vi "Ball&Plate_PID.vi"() -> ()   [LabVIEW 2012]
uses:
  <vilib>/LabVIEW Interface for Arduino/Type Defs/Board Type.ctl
  <vilib>/addons/control/pid/pid.llb/PID (DBL).vi
  <vilib>/LabVIEW Interface for Arduino/LabVIEW Interface for Arduino.lvlib
  <vilib>/vision/NI_Vision_Development_Module.lvlib
  <vilib>/addons/control/pid/NI_PID_pid.lvlib
panel:
  out "Frame Rate":dbl
  out "Posicion actual vs Referencia":cluster{i32[], i32[]}[](graph)
  out "Posicion en el tiempo":cluster{i32, i32}[](graph)
  out "Respuesta en el tiempo":dynamicdata(graph)
  out "Salida PID Y":dbl format="%.2f"
  out "Salida Actuador Y":i32
  out "dt out (s) Y":dbl format="%.3f"
  in  "stop":bool
  in  "Tiempo De Muestreo (ms)":i32
  in  "reinitialize? (F)":bool
  out "dt out (s) X":dbl format="%.3f"
  in  "PID gains":T1={"proportional gain (Kc)"=1.0, "integral time (Ti, min)"=0.01, "derivative time (Td, min)"=0.0} {"derivative time (Td, min)" format="%.3f"; "integral time (Ti, min)" format="%.3f"; "proportional gain (Kc)" format="%.3f"}
  in  "output range":cluster{"output high":dbl, "output low":dbl}={"output high"=100.0, "output low"=-100.0} {"output low" format="%.2f"; "output high" format="%.2f"}
  out "Salida PID X":dbl
  out "ErrorY":dbl
  out "ErrorX":dbl
  in  "Baud Rate (115200)":u32=115200
  in  "Board Type (Uno)":T2
  in  "VISA resource":refnum<visa-resource-name>
  out "Salida Actuador X":i32
  in  "setpoint Y":i32
  in  "setpoint X":i32
  out "Ball and Plate":T3(plugin-control)
  out "POS(X)":i32
  out "POS(Y)":i32
  # "9"
  # "-9"
  # "CONSTANTES"
  # "KP\nKI\nKD"
  # "0,275"
  # "0,375"
  # "0,343"
  # "0,005"
  # "4,985"
  # "0,083"
  # "0,025"
  # "1,256"
  # "0,021"
  # "0,035"
  # "80"
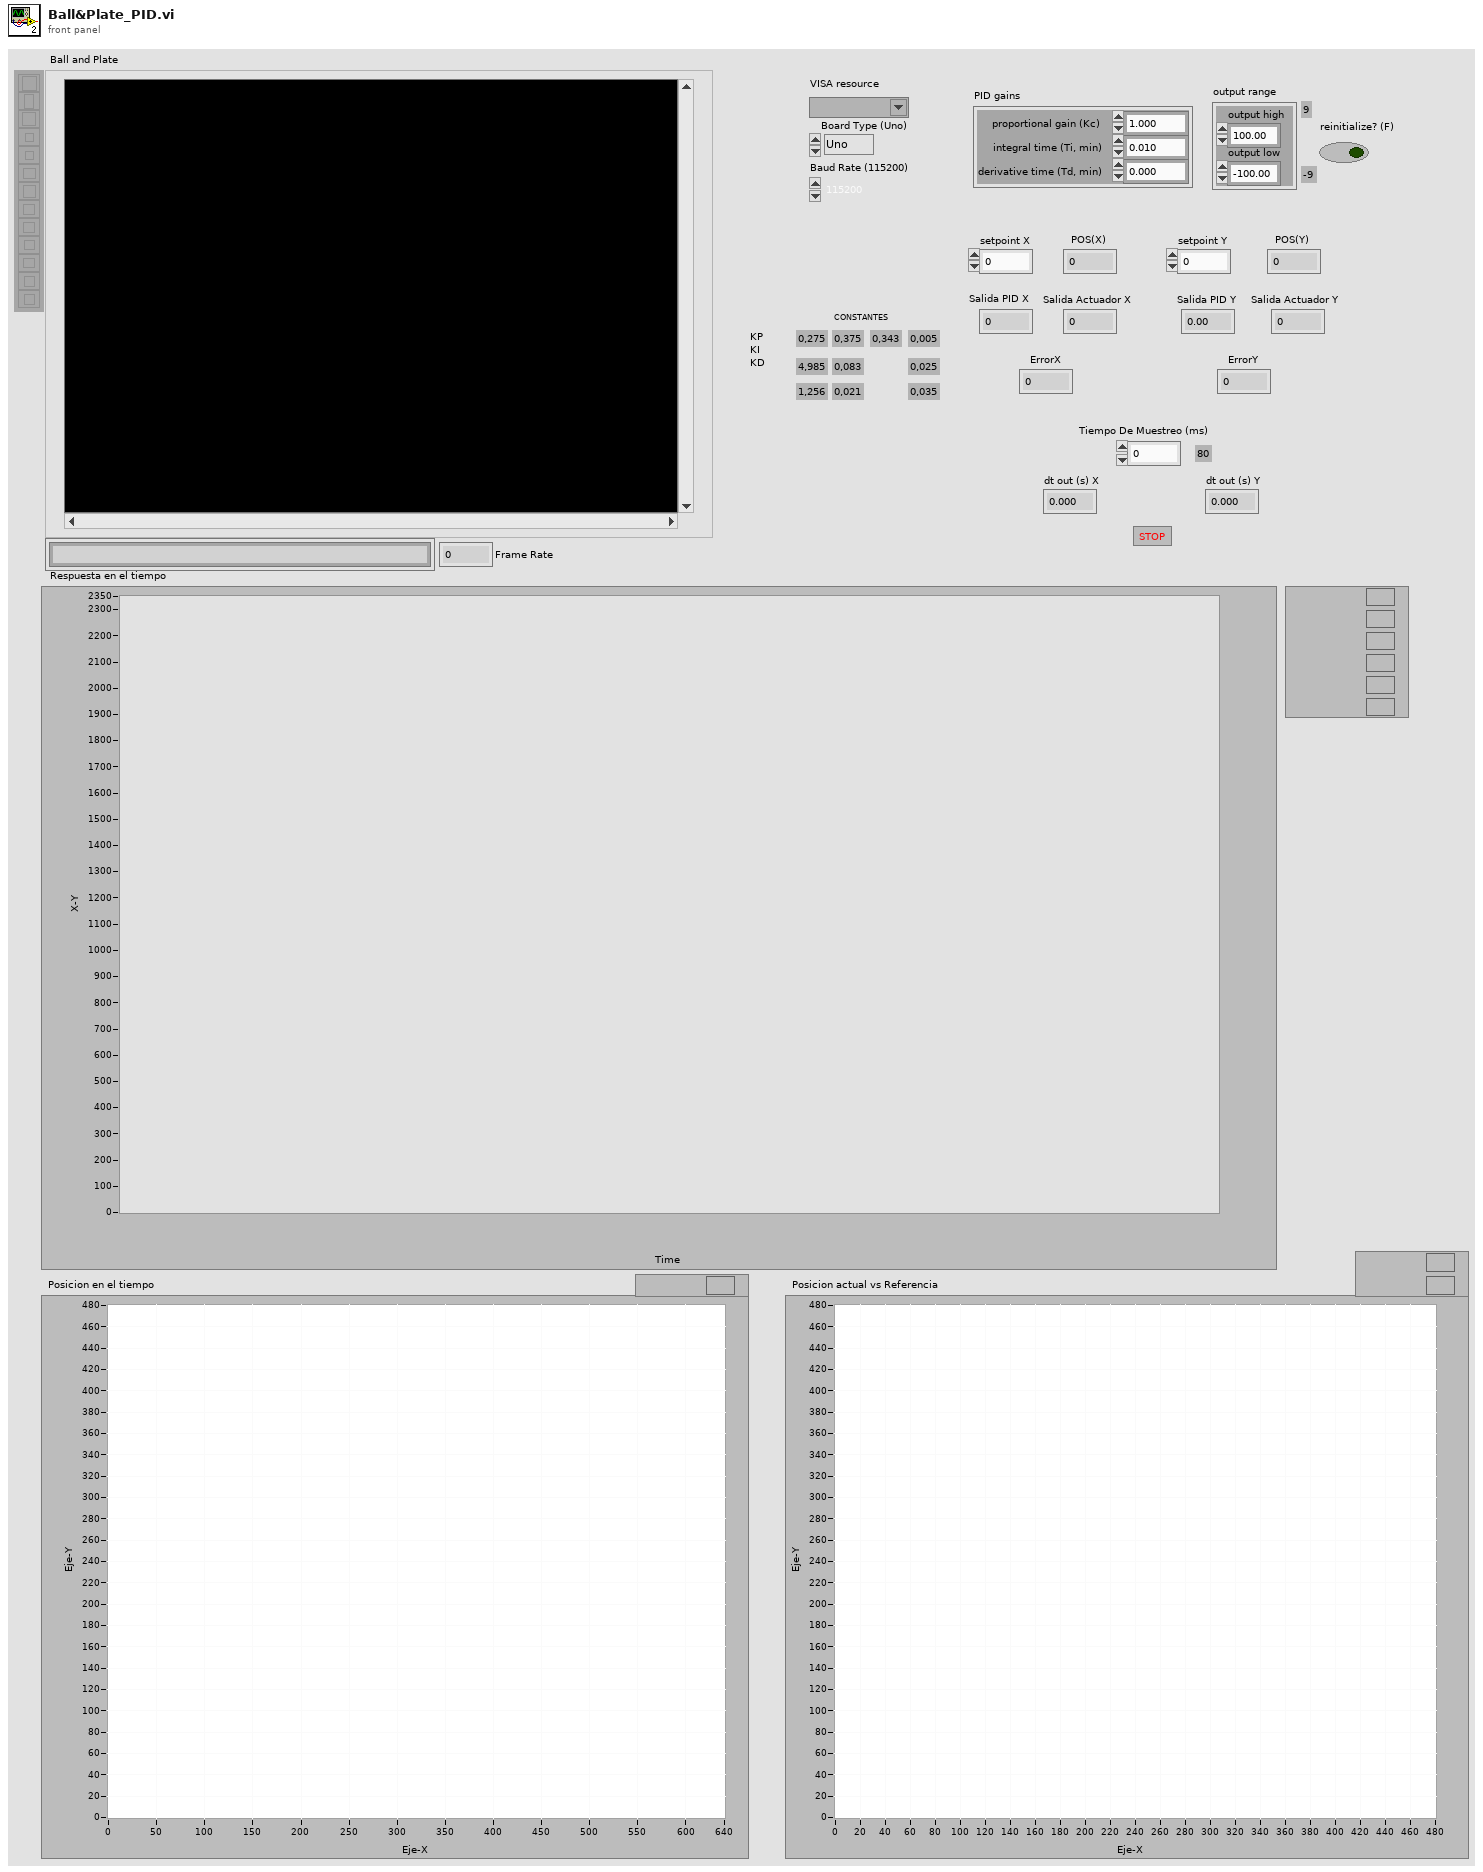
[diagram p1: front panel]
types:
  T1 = cluster{"proportional gain (Kc)":dbl, "integral time (Ti, min)":dbl, "derivative time (Td, min)":dbl}
  T2 = typedef "LabVIEW Interface for Arduino.lvlib/Board Type.ctl" = enum16{"Uno", "Dimuelanove w/Atmega 328", "Mega 2560"}
  T3 = typedef "IMAQ Image.ctl" = refnum<image>
  T4 = typedef "Image Type" = u32
  T5 = typedef "LabVIEW Interface for Arduino.lvlib/Arduino Resource.ctl" = cluster{"VISA resource":refnum<visa-resource-name>, "Board Type":T2, "Connection Type":enum8{"USB / Serial"}, "Bytes Per Packet (15)":u8}
  T6 = cluster{"Position":cluster{"x":sgl, "y":sgl}, "Angle":sgl, "Scale":sgl, "Score":sgl, "Bounding Box":cluster{"x":sgl, "y":sgl}[]}[]
  T7 = cluster{"Matches (Pattern Matching 1)[0]":cluster{"Position":cluster{"x":sgl, "y":sgl}, "Angle":sgl, "Scale":sgl, "Score":sgl, "Bounding Box":cluster{"x":sgl, "y":sgl}[]}, "Matches (Pattern Matching 1)[1]":cluster{"Position":cluster{"x":sgl, "y":sgl}, "Angle":sgl, "Scale":sgl, "Score":sgl, "Bounding Box":cluster{"x":sgl, "y":sgl}[]}, "Matches (Pattern Matching 1)[2]":cluster{"Position":cluster{"x":sgl, "y":sgl}, "Angle":sgl, "Scale":sgl, "Score":sgl, "Bounding Box":cluster{"x":sgl, "y":sgl}[]}, "Matches (Pattern Matching 1)[3]":cluster{"Position":cluster{"x":sgl, "y":sgl}, "Angle":sgl, "Scale":sgl, "Score":sgl, "Bounding Box":cluster{"x":sgl, "y":sgl}[]}}
  T8 = cluster{"Bounding Box[0]":cluster{"x":sgl, "y":sgl}, "Bounding Box[1]":cluster{"x":sgl, "y":sgl}, "Bounding Box[2]":cluster{"x":sgl, "y":sgl}, "Bounding Box[3]":cluster{"x":sgl, "y":sgl}}
  T9 = cluster{"[0]":sgl, "[1]":sgl, "[2]":sgl, "[3]":sgl}
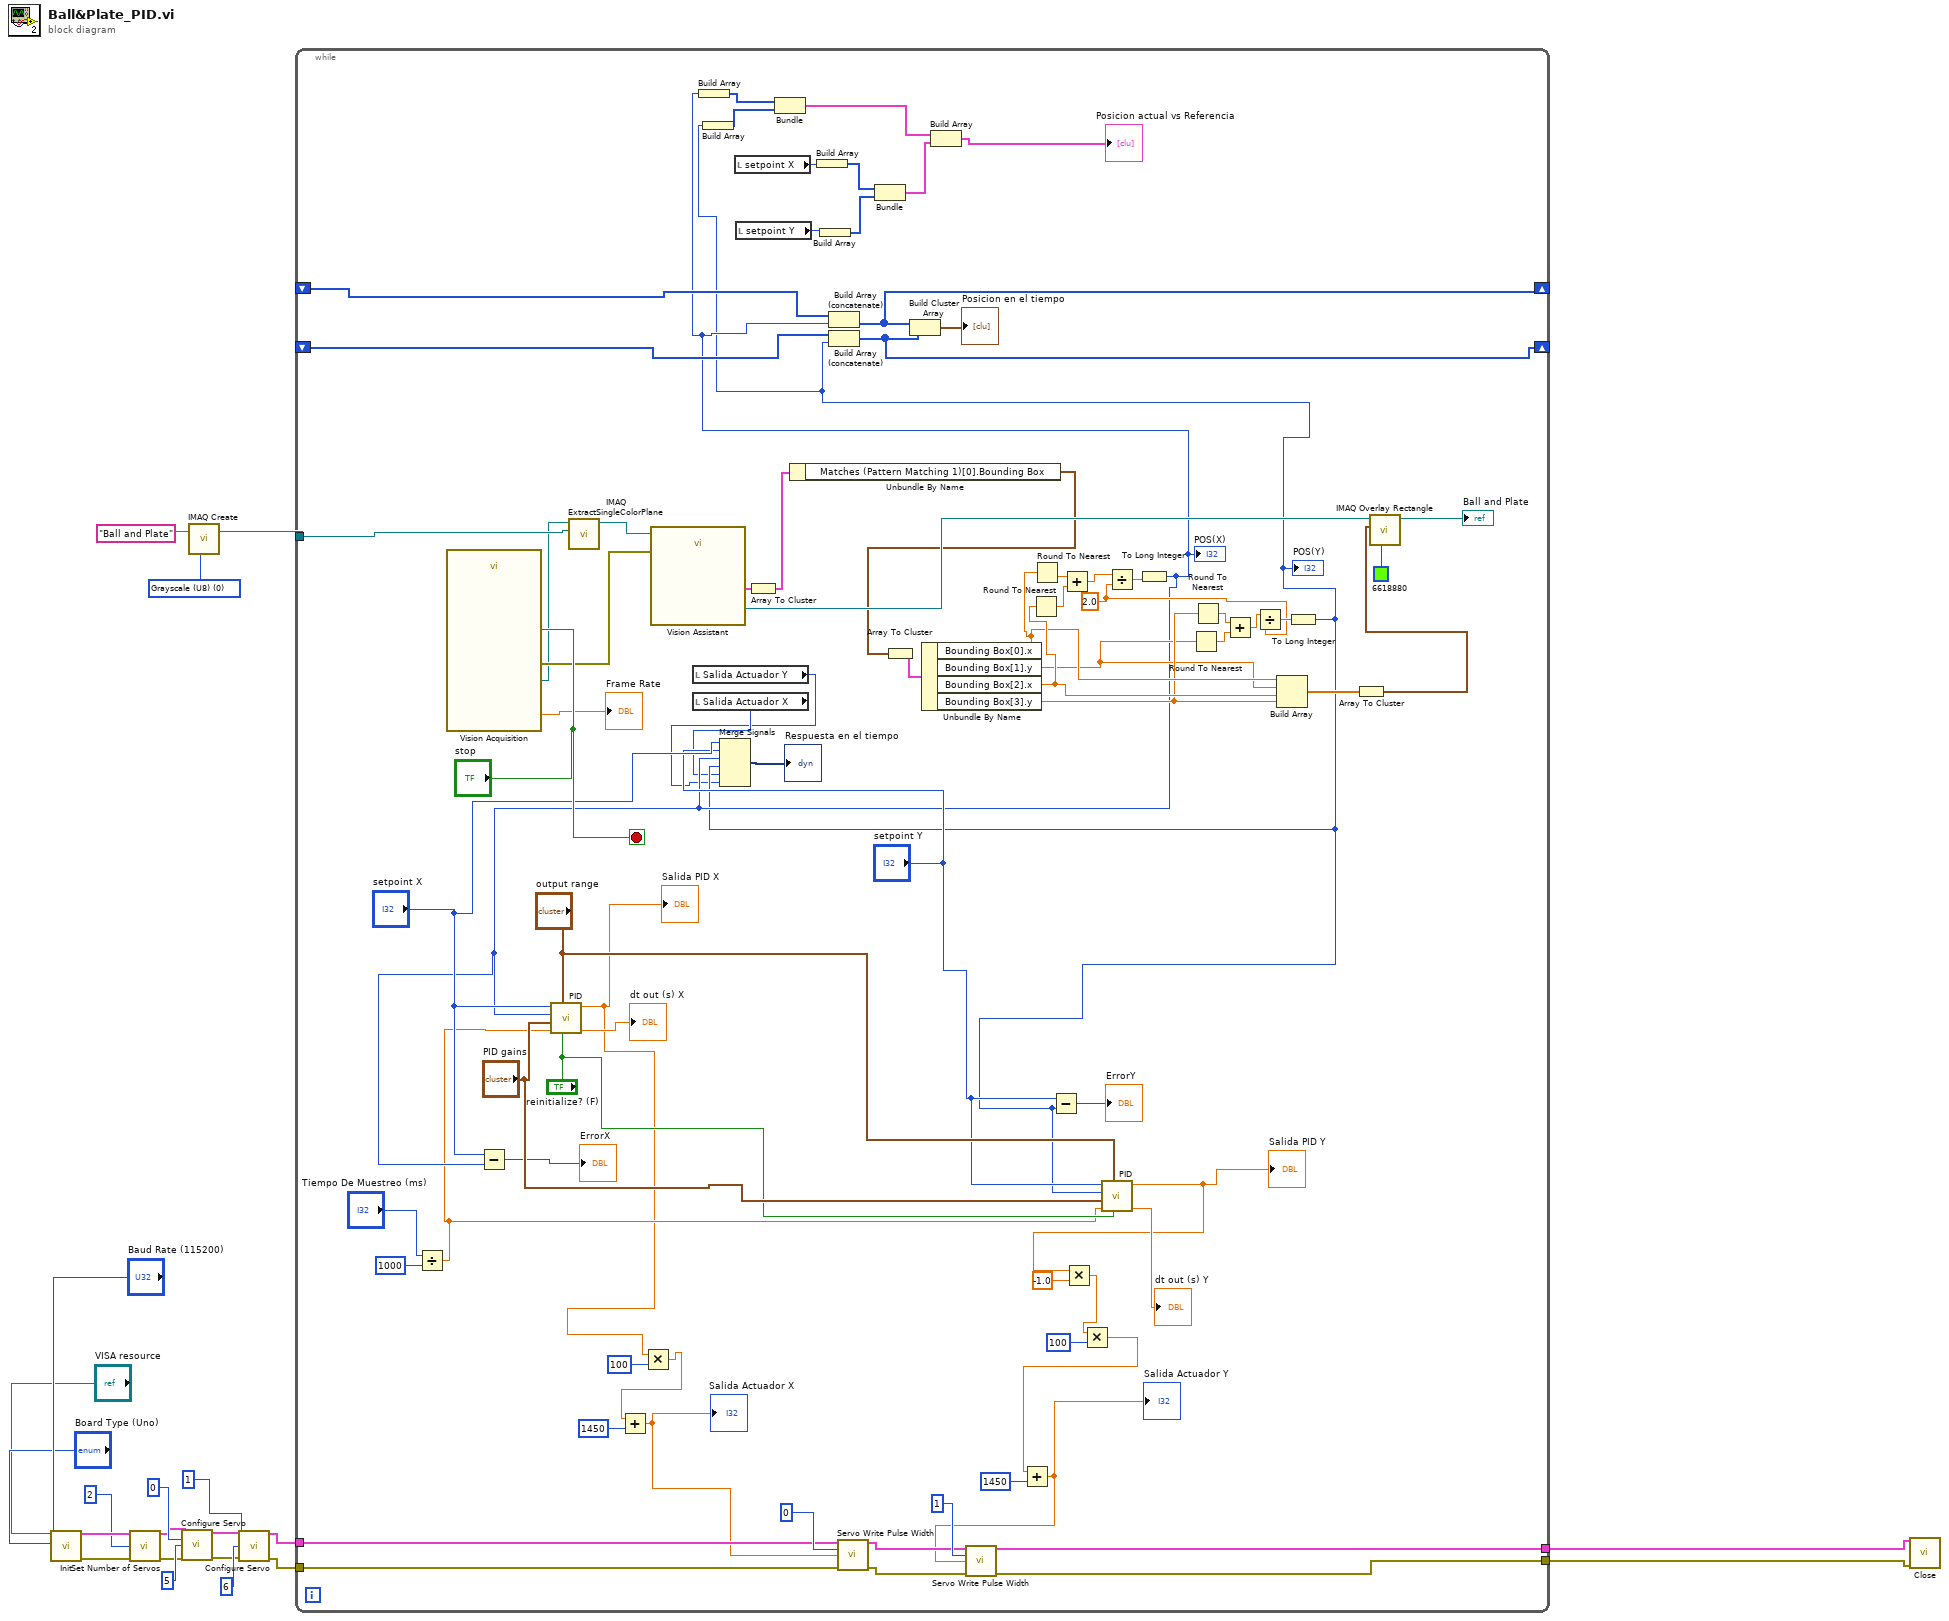
[diagram p0: block diagram]
diagram:
  w21 = T4 0 items=["Grayscale (U8)", "Grayscale (I16)", "Grayscale (SGL)", "Complex (CSG)", "RGB (U32)", "HSL (U32)", "RGB (U64)", "Grayscale (U16)"] ("Image Type")
  n1 = call <vilib>:"Init.vi"("VISA resource"="VISA resource", "Baud Rate (115200)"="Baud Rate (115200)", "Board Type (Uno)"="Board Type (Uno)") -> ("Arduino Resource"=w9:T5, "error out"=w8:errorcluster)  [unwired: 15 in]
  n2 = call <vilib>:"Set Number of Servos.vi"("Arduino Resource"=w9, "Number Of Servos (1)"=u8 2, "error in"=w8) -> ("Arduino Resource"=w10:T5, "error out"=w12:errorcluster)  [unwired: 11 in]
  n3 = call <vilib>:"Configure Servo.vi"("Arduino Resource"=w10, "Servo Number (0)"=u8 0, "DIO Pin (2)"=u8 5, "error in"=w12) -> ("Arduino Resource"=w11:T5, "error out"=w13:errorcluster)  [unwired: 10 in]
  n4 = call "IMAQ Create"("Image Name"="Ball and Plate", "Image Type"=w21) -> ("New Image"=w3:T3)  [unwired: 3 in, 1 out]
  n5 = call <vilib>:"Configure Servo.vi"("Arduino Resource"=w11, "Servo Number (0)"=u8 1, "DIO Pin (2)"=u8 6, "error in"=w13) -> ("Arduino Resource"=w5:T5, "error out"=w4:errorcluster)  [unwired: 10 in]
  n6 = while {
    tunnel: w5 -> [w95]
    tunnel: w4 -> [w94]
    tunnel: [w93] -> w2
    tunnel: w3 -> [w92]
    tunnel: [w58] -> w1
    shift-right: [w56] -> _
    shift-left: _ -> [w54]
    shift-right: [w55] -> _
    shift-left: _ -> [w53]
    stop <- "stop" stop-if-true
    w66 = sgl 2.0 ("x")
    n7 = Divide(x="Tiempo De Muestreo (ms)", y=1000) -> (x/y=w39:dbl)
    n8 = call "Vision Acquisition"("Stop (F)"="stop") -> ("Image Out"=w68:T3, "Frame Rate"=→"Frame Rate":dbl, "error out"=w75:errorcluster)  [unwired: 23 in, 1 out]
    n9 = call "IMAQ ExtractSingleColorPlane"("Image Dst"=w92, "Image Src"=w68) -> ("Image Dst Out"=w74:T3)  [unwired: 8 in, 1 out]
    n10 = call "Vision Assistant"("Image In"=w74, "error in"=w75) -> ("Image Out"=w77:T3, "Matches (Pattern Matching 1)"=w76:T6)  [unwired: 23 in, 1 out]
    n11 = local read "Salida Actuador Y"() -> (w26:i32)
    n12 = local read "Salida Actuador X"() -> (w27:i32)
    n13 = local read "setpoint X"() -> (w43:i32)
    n14 = local read "setpoint Y"() -> (w42:i32)
    n15 = Array To Cluster(array=w76) -> (cluster=w79:T7)
    n16 = Unbundle By Name(w79) -> ("Matches (Pattern Matching 1)[0].Bounding Box"=w71:cluster{"x":sgl, "y":sgl}[])
    n17 = Build Array(w43) -> (w52:i32[])
    n18 = Build Array(w42) -> (w51:i32[])
    n19 = Bundle(w52, w51) -> (w46:cluster{i32[], i32[]})  [unwired: 1 in]
    n20 = Array To Cluster ("Array To Cluster 2")(array=w71) -> (cluster=w72:T8)
    n21 = Unbundle By Name ("Unbundle By Name 2")(w72) -> ("Bounding Box[0].x"=w88:sgl, "Bounding Box[1].y"=w82:sgl, "Bounding Box[2].x"=w89:sgl, "Bounding Box[3].y"=w83:sgl)
    n22 = Round To Nearest(number=w89) -> (nearest integer value=w87:sgl)
    n23 = Round To Nearest ("Round To Nearest 3")(number=w88) -> (nearest integer value=w86:sgl)
    n24 = Add ("Add 2")(x=w86, y=w87) -> (x+y=w90:sgl)
    n25 = Divide(x=w90, y=w66) -> (x/y=w69:sgl)
    n26 = To Long Integer(number=w69) -> (32bit integer=w45:i32)
    "POS(X)" <- w45
    n27 = Subtract(x="setpoint X", y=w45) -> (x-y=→"ErrorX":i32)
    n28 = call-poly <vilib>:"PID.vi"("reinitialize? (F)"="reinitialize? (F)", "output range"="output range", "dt (s)"=w39, "PID gains"="PID gains", "process variable"=w45, "setpoint"="setpoint X") -> ("dt out (s)"=→"dt out (s) X":dbl, "output"=w36:dbl)  [unwired: 4 in]
    "Salida PID X" <- w36
    n29 = Multiply(x=w36, y=100) -> (x*y=w32:dbl)
    n30 = Add(x=w32, y=1450) -> (x+y=w23:dbl)
    "Salida Actuador X" <- w23
    n31 = Build Array(w45) -> (w50:i32[])
    n32 = Build Array (concatenate)(w54, w45) -> (w56:i32[])
    n33 = call <vilib>:"Servo Write Pulse Width.vi"("Arduino Resource"=w95, "Servo Number"=u8 0, "Pulse Width in uS"=w23, "error in"=w94) -> ("Arduino Resource"=w96:T5, "error out"=w97:errorcluster)  [unwired: 10 in]
    n34 = Round To Nearest ("Round To Nearest 2")(number=w82) -> (nearest integer value=w85:sgl)
    n35 = Round To Nearest ("Round To Nearest 4")(number=w83) -> (nearest integer value=w84:sgl)
    n36 = Add(x=w84, y=w85) -> (x+y=w67:sgl)
    n37 = Divide ("Divide 2")(x=w67, y=w66) -> (x/y=w70:sgl)
    n38 = Build Array(w88, w82, w89, w83) -> (w80:sgl[])
    n39 = To Long Integer(number=w70) -> (32bit integer=w44:i32)
    "POS(Y)" <- w44
    n40 = Build Array(w44) -> (w49:i32[])
    n41 = Merge Signals("setpoint X", "setpoint Y", w45, w44, w27, w26) -> (→"Respuesta en el tiempo":dynamicdata)
    n42 = Bundle(w50, w49) -> (w47:cluster{i32[], i32[]})  [unwired: 1 in]
    n43 = Build Array (concatenate)(w53, w44) -> (w55:i32[])
    n44 = Build Cluster Array(w56, w55) -> (→"Posicion en el tiempo":cluster{i32, i32}[])
    n45 = Build Array(w47, w46) -> (→"Posicion actual vs Referencia":cluster{i32[], i32[]}[])
    n46 = Subtract ("Subtract 2")(x="setpoint Y", y=w44) -> (x-y=→"ErrorY":i32)
    n47 = call-poly <vilib>:"PID.vi"("reinitialize? (F)"="reinitialize? (F)", "output range"="output range", "dt (s)"=w39, "PID gains"="PID gains", "process variable"=w44, "setpoint"="setpoint Y") -> ("dt out (s)"=→"dt out (s) Y":dbl, "output"=w30:dbl)  [unwired: 4 in]
    "Salida PID Y" <- w30
    n48 = Multiply(x=w30, y=-1.0) -> (x*y=w28:dbl)
    n49 = Multiply(x=w28, y=100) -> (x*y=w31:dbl)
    n50 = Add(x=w31, y=1450) -> (x+y=w22:dbl)
    "Salida Actuador Y" <- w22
    n51 = call <vilib>:"Servo Write Pulse Width.vi"("Arduino Resource"=w96, "Servo Number"=u8 1, "Pulse Width in uS"=w22, "error in"=w97) -> ("Arduino Resource"=w93:T5, "error out"=w58:errorcluster)  [unwired: 10 in]
    n52 = Array To Cluster ("Array To Cluster 3")(array=w80) -> (cluster=w81:T9)
    n53 = call "IMAQ Overlay Rectangle"("Color"=u32 6618880, "Rectangle"=w81, "Image"=w77) -> ("Image Out"=→"Ball and Plate":T3)  [unwired: 7 in, 1 out]
  }
  n54 = call <vilib>:"Close.vi"("Arduino Resource"=w2, "error in"=w1) -> ()  [unwired: 13 in, 1 out]
